vi "Write Property.vi"(6 "timeout (ms)":i32=-1, 8 "error in (no error)":errorcluster, 9 "Property Value":string, 10 "Property Name":string, 11 "FlexLogger_gRPCAPI in":refnum<class "FlexLogger_gRPC.lvclass">) -> (0 "error out":errorcluster, 3 "FlexLogger_gRPCAPI out":refnum<class "FlexLogger_gRPC.lvclass">)   [LabVIEW 2020, in "FlexLogger_gRPC.lvlib" / "FlexLogger_gRPC.lvclass"]
doc: "Sets a specific test property of currently opened project in flexlogger"
uses:
  FlexLogger_gRPC.lvclass
  FlexLogger_client/RPC Messages/flexlogger_SetTestPropertyRequest.ctl
  FlexLogger_client/RPC Messages/flexlogger_ElementIdentifier.ctl
  FlexLogger_client/RPC Messages/flexlogger_TestProperty.ctl
  FlexLogger_gRPC.lvclass/FlexLogger_gRPC.ctl
  FlexLogger_client/FlexLogger_client.lvlib
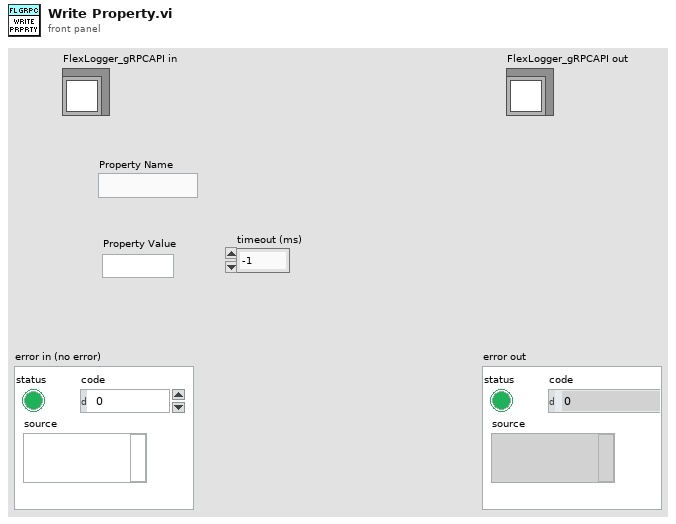
[diagram p1: front panel]
types:
  T1 = typedef "FlexLogger_client.lvlib/flexlogger_SetTestPropertyRequest.ctl" = cluster{"document_identifier":T2, "test_property":T3}
  T2 = typedef "FlexLogger_client.lvlib/flexlogger_ElementIdentifier.ctl" = cluster{"project_id":string, "file_name":string, "element_id":string, "subpart_id":string}
  T3 = typedef "FlexLogger_client.lvlib/flexlogger_TestProperty.ctl" = cluster{"property_name":string, "property_value":string, "prompt_on_start":bool}
  T4 = typedef "grpc-lvsupport-release.lvlib/grpcId.ctl" = u64
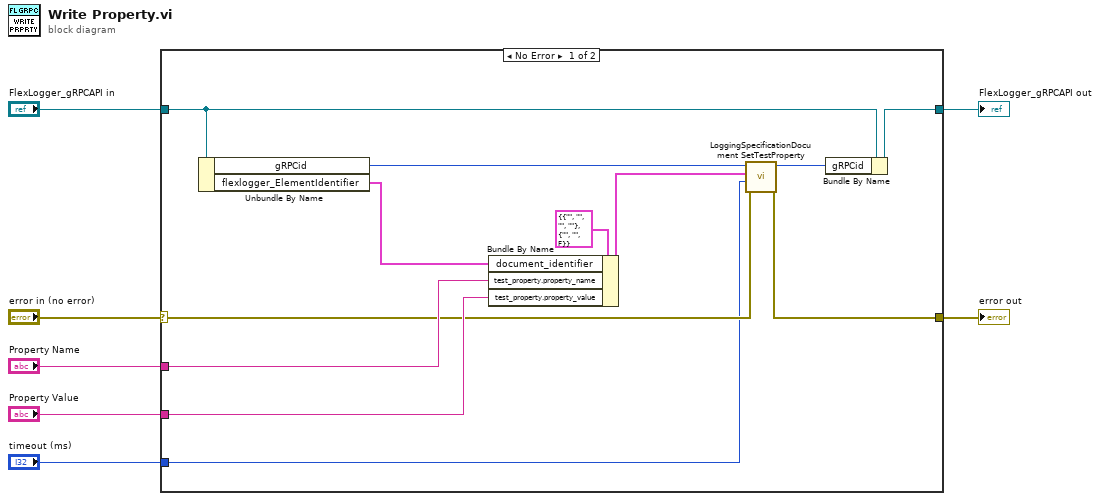
[diagram p0: block diagram]
diagram:
  n1 = case shown="No Error" "error in (no error)" {
    selector: "error in (no error)" -> [w9 w20]
    tunnel: "FlexLogger_gRPCAPI in" -> [w19 w21]
    tunnel: [w18 w21] -> w7
    tunnel: [w16 w20] -> w6
    tunnel: "Property Name" -> [w14 _]
    tunnel: "Property Value" -> [w12 _]
    tunnel: "timeout (ms)" -> [w8 _]
    frame No Error {
      n2 = Unbundle By Name(w19) -> ("gRPCid"=w11:T4, "flexlogger_ElementIdentifier"=w10:T2)
      n3 = Bundle By Name(cluster=T1 {"document_identifier"={"project_id"="", "file_name"="", "element_id"="", "subpart_id"=""}, "test_property"={"property_name"="", "property_value"="", "prompt_on_start"=FALSE}} ("Request Data"), "document_identifier"=w10, "test_property.property_name"=w14, "test_property.property_value"=w12) -> (w13:T1)
      n4 = call "LoggingSpecificationDocument SetTestProperty.vi"("error in"=w9, "timeout (ms)"=w8, "Request Data"=w13, "gRPC ID"=w11) -> ("error out"=w16:errorcluster, "gRPC ID out"=w17:T4)  [unwired: 5 in, 1 out]
      n5 = Bundle By Name(cluster=w19, "gRPCid"=w17) -> (w18:refnum<class "FlexLogger_gRPC.lvclass">)
    }
    frame Error {
    }
  }
  "error out" <- w6
  "FlexLogger_gRPCAPI out" <- w7
